vi "myrio_usb_info.vi"(10 "Path":path=path "u:/") -> (0 "Free Capacity [%]":u8, 1 "Free Capacity [MB]":u32, 2 "Total Capacity [MB]":u32, 3 "USB flash drive info":string, 4 "filenames":string[](array[string]), 6 "folder names":string[](array[string]))   [LabVIEW 2019]
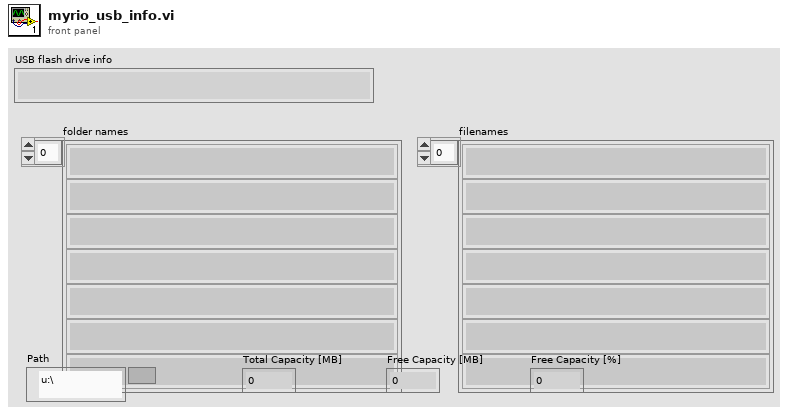
[diagram p1: front panel]
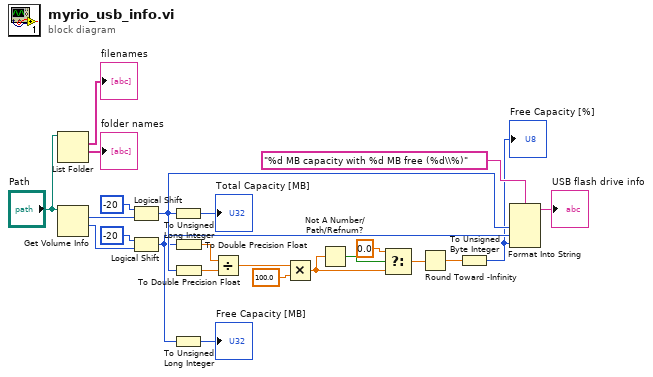
[diagram p0: block diagram]
diagram:
  n1 = List Folder(path="Path") -> (filenames=→"filenames":string[], folder names=→"folder names":string[])  [unwired: 3 in, 2 out]
  n2 = Get Volume Info(11:"Path") -> (1:w20:i64, 2:w21:i64)  [unwired: 1 in, 4 out]
  n3 = Logical Shift(y=i16 -20, x=w21) -> (x << y=w7:i64)
  n4 = Logical Shift(y=i16 -20, x=w20) -> (x << y=w5:i64)
  n5 = To Unsigned Long Integer(number=w7) -> (unsigned 32bit integer=→"Total Capacity [MB]":u32)
  n6 = To Unsigned Long Integer(number=w5) -> (unsigned 32bit integer=→"Free Capacity [MB]":u32)
  n7 = To Double Precision Float(number=w5) -> (double precision float=w17:dbl)
  n8 = To Double Precision Float(number=w7) -> (double precision float=w16:dbl)
  n9 = Divide(x=w17, y=w16) -> (x/y=w12:dbl)
  n10 = Multiply(x=w12, y=100.0) -> (x*y=w9:dbl)
  n11 = Not A Number/Path/Refnum?(number/path/refnum=w9) -> (NaN/Path/Refnum?=w10:bool)
  n12 = Select(t=0.0, s=w10, f=w9) -> (s? t:f=w2:dbl)
  n13 = Round Toward -Infinity(1:w2) -> (0:w1:dbl)
  n14 = To Unsigned Byte Integer(number=w1) -> (unsigned 8bit integer=w3:u8)
  "Free Capacity [%]" <- w3
  n15 = Format Into String(format string="%d MB capacity with %d MB free (%d\\%)", w7, w5, w3) -> (resulting string=→"USB flash drive info":string)  [unwired: 2 in, 1 out]
